vi "matlab_TI2_shutter.vi"(8 "error in":errorcluster, 10 "Shutter":bool=TRUE) -> (0 "error out":errorcluster)   [LabVIEW 2018]
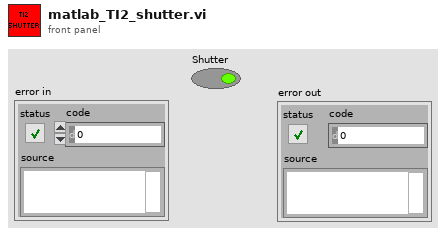
[diagram p1: front panel]
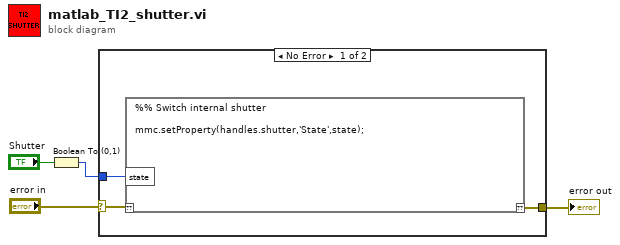
[diagram p0: block diagram]
diagram:
  n1 = Boolean To (0,1)(Boolean="Shutter") -> (0, 1=w2:i16)
  n2 = case shown="No Error" "error in" {
    selector: "error in" -> [w7 w8]
    tunnel: [w6 w8] -> w3
    tunnel: w2 -> [w5 _]
    frame No Error {
      n3 = script code="%% Switch internal shutter\n\nmmc.setProperty(handles.shutter,'State',state);"("??"=w7, "state"=w5) -> ("??"=w6:errorcluster)
    }
    frame Error {
    }
  }
  "error out" <- w3
